vi "RW Manual Ctrl.vi"() -> ()   [LabVIEW 2012]
uses:
  <vilib>/Instr/_visa.llb/VISA Configure Serial Port (Instr).vi
panel:
  out "cos function":dbl
  in  "bytes to read":u32=12
  out "bytes read":u32
  out "CMD code":string
  in  "Control Value":sgl=1.0 format="%.4f"
  out "init":string
  out "ping":string
  in  "Amplitude":dbl
  in  "Frequency":dbl
  in  "STOP":bool caption="stop (F)"
  in  "Dst":i32=54 format="%x"
  in  "Control Mode":u16(ring) items=["Idle"=0, "PWM (-1..1)"=1, "Current (-2.5..2.5A)"=2, "Speed (Rads/s)"=3, "Acceleration (Rads/sec^2)"=16, "Momentum (N-m-sec)"=17, "Torque (N-m)"=18]
  out "bytes written":u32
  out "Read string":string
  in  "VISA resource name (write)":refnum<visa-resource-name>="COM4"
  in  "Reaction Wheel":bool
  in  "stop bits":u16(ring)=10 items=["1.0"=10, "1.5"=15, "2.0"=20]
  in  "flow control":u16(ring) items=["None"=0, "XON/XOFF"=1, "RTS/CTS"=2, "DTR/DSR"=4]
  in  "parity (0:none)":u16(ring) items=["None", "Odd", "Even", "Mark", "Space"]
  in  "data bits (8)":u16=8 min=5 max=8 step=1
  in  "baud rate (115200)":u32=115200
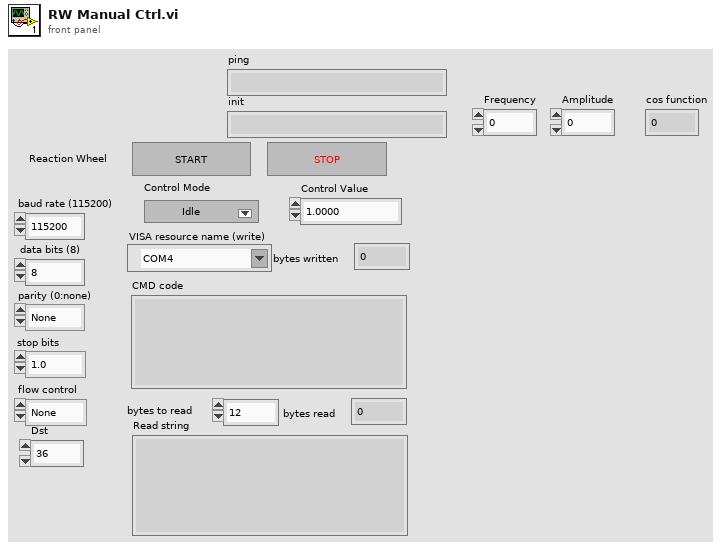
[diagram p1: front panel]
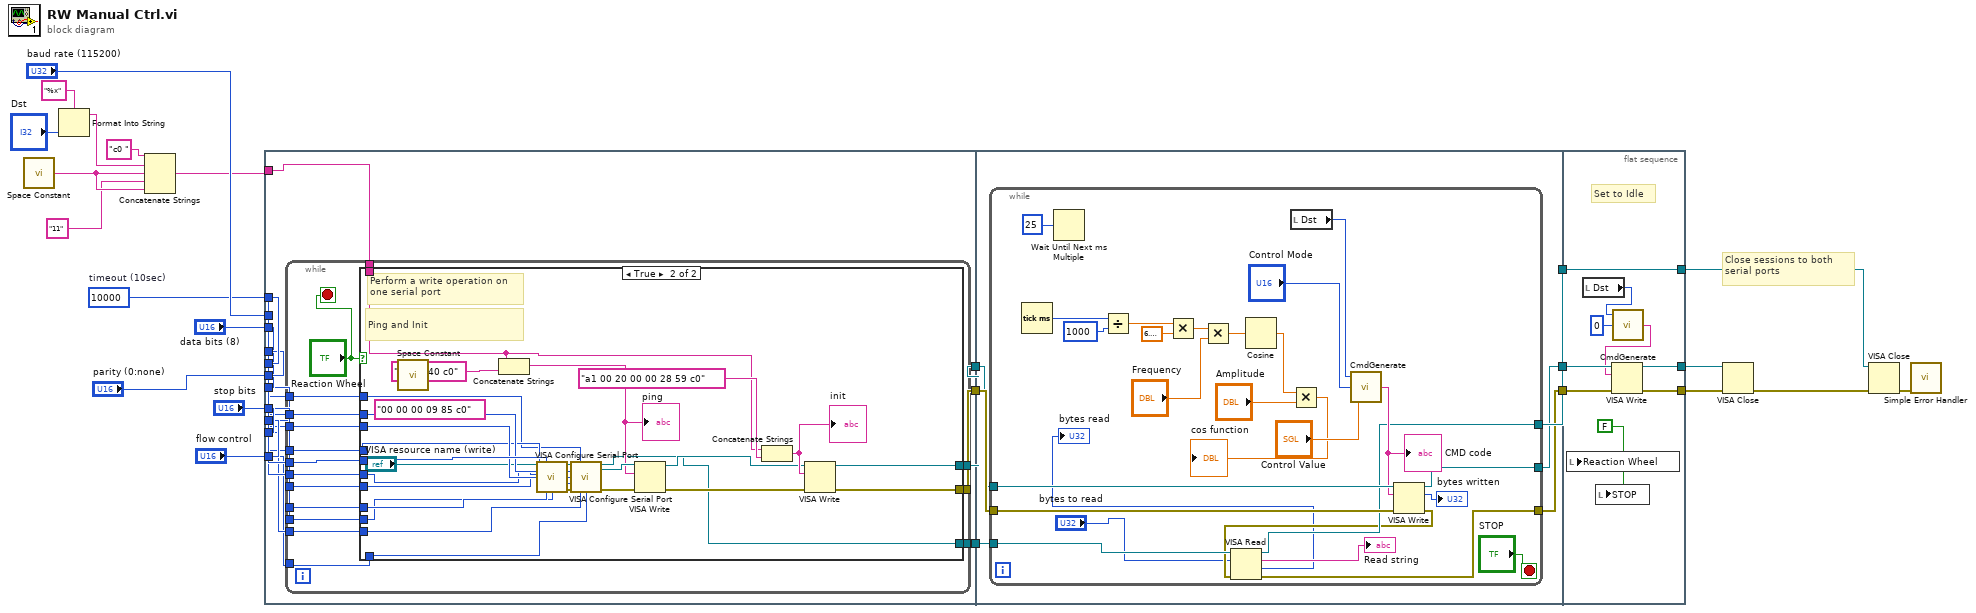
[diagram p0: block diagram]
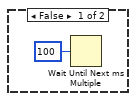
[diagram p2: hidden frame]
diagram:
  w11 = u32 10000  # timeout (10sec)
  # "Close sessions to both serial ports"
  n1 = call <vilib>:"Space Constant.vi"() -> ("String"=w13:string)
  n2 = Format Into String(format string="%x", "Dst") -> (resulting string=w14:string)  [unwired: 2 in, 1 out]
  n3 = Concatenate Strings("c0 " ("string"), w14, w13, "11", w13) -> (w6:string)
  n4 = flat-sequence {
    tunnel: [w39] -> w24
    tunnel: [w38] -> w23
    tunnel: w11 -> [w37]
    tunnel: "stop bits" -> [w36]
    tunnel: "flow control" -> [w35]
    tunnel: "baud rate (115200)" -> [w34]
    tunnel: "data bits (8)" -> [w33]
    tunnel: "parity (0:none)" -> [w32]
    tunnel: w11 -> [w31]
    tunnel: "parity (0:none)" -> [w30]
    tunnel: "data bits (8)" -> [w29]
    tunnel: "stop bits" -> [w28]
    tunnel: "flow control" -> [w27]
    tunnel: w6 -> [w26]
    tunnel: [w25] -> w3
    tunnel: w24 -> [w82]
    tunnel: w23 -> [w86]
    tunnel: [w87] -> w22
    tunnel: [w85] -> w21
    tunnel: [w84] -> w20
    tunnel: w3 -> [w83]
    tunnel: [w121] -> w4
    tunnel: [w120] -> w5
    tunnel: [w123] -> w17
    tunnel: w22 -> [w123]
    tunnel: w21 -> [w119]
    tunnel: w20 -> [w122]
    frame #0 {
      n5 = while {
        tunnel: [w55] -> w39
        tunnel: [w54] -> w38
        tunnel: w37 -> [w53]
        tunnel: w36 -> [w52]
        tunnel: w35 -> [w51]
        tunnel: w34 -> [w50]
        tunnel: w33 -> [w49]
        tunnel: w32 -> [w48]
        tunnel: w31 -> [w47]
        tunnel: w30 -> [w46]
        tunnel: w29 -> [w45]
        tunnel: w28 -> [w44]
        tunnel: w27 -> [w43]
        tunnel: w26 -> [w42]
        tunnel: [w40] -> w25
        stop <- "Reaction Wheel" stop-if-true
        n6 = case shown="True" "Reaction Wheel" {
          tunnel: [_ w75] -> w55
          tunnel: [_ w74] -> w54
          tunnel: w53 -> [_ w73]
          tunnel: w52 -> [_ w72]
          tunnel: w51 -> [_ w71]
          tunnel: w50 -> [_ w70]
          tunnel: w49 -> [_ w69]
          tunnel: w48 -> [_ w68]
          tunnel: w47 -> [_ w67]
          tunnel: w46 -> [_ w66]
          tunnel: w45 -> [_ w65]
          tunnel: w44 -> [_ w64]
          tunnel: w43 -> [_ w63]
          tunnel: w42 -> [_ w60]
          tunnel: [_ w57] -> w40
          frame False {
            n7 = Wait Until Next ms Multiple(millisecond multiple=u32 100) -> ()  [unwired: 1 out]
          }
          frame True {
            (unwired) "00 00 00 09 85 c0"
            # "Perform a write operation on one serial port"
            # "Ping and Init"
            n8 = call <vilib>:"Space Constant.vi"() -> ()  [unwired: 1 out]
            n9 = Concatenate Strings(w60, "a0 07 40 c0" ("string")) -> (w61:string)
            "ping" <- w61
            n10 = call-poly "VISA Configure Serial Port"("VISA resource name"="VISA resource name (write)", "timeout (10sec)"=w73, "baud rate (9600)"=w66, "data bits (8)"=w65, "stop bits (10: 1 bit)"=w72, "flow control (0:none)"=w71) -> ("VISA resource name out"=w76:refnum<visa-resource-name>, "error out"=w77:errorcluster)  [unwired: 3 in, 5 out]
            n11 = call-poly "VISA Configure Serial Port"("VISA resource name"="VISA resource name (write)", "timeout (10sec)"=w67, "baud rate (9600)"=w70, "data bits (8)"=w69, "parity (0:none)"=w68, "error in (no error)"=w77, "stop bits (10: 1 bit)"=w64, "flow control (0:none)"=w63) -> ("VISA resource name out"=w57:refnum<visa-resource-name>, "error out"=w78:errorcluster)  [unwired: 2 in, 4 out]
            n12 = VISA Write(VISA resource name=w76, write buffer=w61, error in (no error)=w78) -> (VISA resource name out=w79:refnum<visa-resource-name>, error out=w58:errorcluster)  [unwired: 1 out]
            n13 = Concatenate Strings(w60, "a1 00 20 00 00 28 59 c0" ("string")) -> (w81:string)
            "init" <- w81
            n14 = VISA Write(VISA resource name=w79, write buffer=w81, error in (no error)=w58) -> (VISA resource name out=w75:refnum<visa-resource-name>, error out=w74:errorcluster)  [unwired: 1 out]
          }
        }
      }
    }
    frame #1 {
      n15 = while {
        tunnel: [w94] -> w87
        tunnel: w82 -> [w114]
        tunnel: w86 -> [w113]
        tunnel: [w92] -> w85
        tunnel: [w112] -> w84
        tunnel: w83 -> [w95]
        stop <- "STOP" stop-if-true
        n16 = Tick Count (ms)() -> (millisecond timer value=w105:u32)
        n17 = Wait Until Next ms Multiple(millisecond multiple=u32 25) -> ()  [unwired: 1 out]
        n18 = Divide(x=w105, y=1000) -> (x/y=w103:dbl)
        n19 = Multiply(x=w103, y=6.283185307179586) -> (x*y=w101:dbl)
        n20 = Multiply(x=w101, y="Frequency") -> (x*y=w99:dbl)
        n21 = Cosine(x=w99) -> (cos(x)=w98:dbl)
        n22 = local read "Dst"() -> (w111:i32)
        n23 = Multiply(x=w98, y="Amplitude") -> (x*y=→"cos function":dbl)
        n24 = call "CmdGenerate.vi"("Control Value"="Control Value", "Mode"="Control Mode", "Dst"=w111) -> ("CMD code"=w108:string)
        "CMD code" <- w108
        n25 = VISA Write(VISA resource name=w114, write buffer=w108, error in (no error)=w113) -> (VISA resource name out=w112:refnum<visa-resource-name>, return count=→"bytes written":u32, error out=w93:errorcluster)
        n26 = VISA Read(VISA resource name=w95, byte count="bytes to read", error in (no error)=w93) -> (VISA resource name out=w94:refnum<visa-resource-name>, read buffer=→"Read string":string, return count=→"bytes read":u32, error out=w92:errorcluster)
      }
    }
    frame #2 {
      w115 = FALSE
      # "Set to Idle"
      n27 = local write "Reaction Wheel"(w115) -> ()
      n28 = local read "Dst"() -> (w118:i32)
      n29 = local write "STOP"(w115) -> ()
      n30 = call "CmdGenerate.vi"("Mode"=0, "Dst"=w118) -> ("CMD code"=w116:string)  [unwired: 1 in]
      n31 = VISA Write(VISA resource name=w122, write buffer=w116, error in (no error)=w119) -> (VISA resource name out=w121:refnum<visa-resource-name>, error out=w120:errorcluster)  [unwired: 1 out]
    }
  }
  n32 = VISA Close(VISA resource name=w4, error in (no error)=w5) -> (error out=w19:errorcluster)
  n33 = VISA Close(VISA resource name=w17, error in (no error)=w19) -> (error out=w18:errorcluster)
  n34 = call <vilib>:"Simple Error Handler.vi"("error in (no error)"=w18) -> ()  [unwired: 1 in, 8 out]
